vi "TankFill.vi"() -> ()   [LabVIEW 2018]
panel:
  out "?":string
  out "Min. Level":bool
  out "Max. Level":bool
  in  "Decrement/0.1sec":dbl(knob) scale=0.0..10.0
  in  "Increment/0.1sec":dbl(knob) scale=0.0..10.0
  in  "Min level":dbl(knob) scale=0.0..100.0
  in  "Max level":dbl(knob) scale=0.0..100.0
  out "Tank":dbl(slide) scale=0.0..100.0
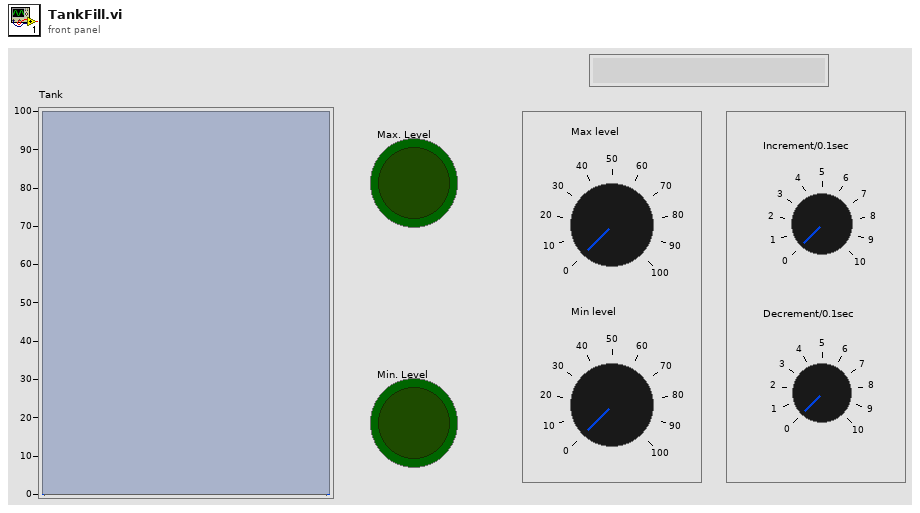
[diagram p1: front panel]
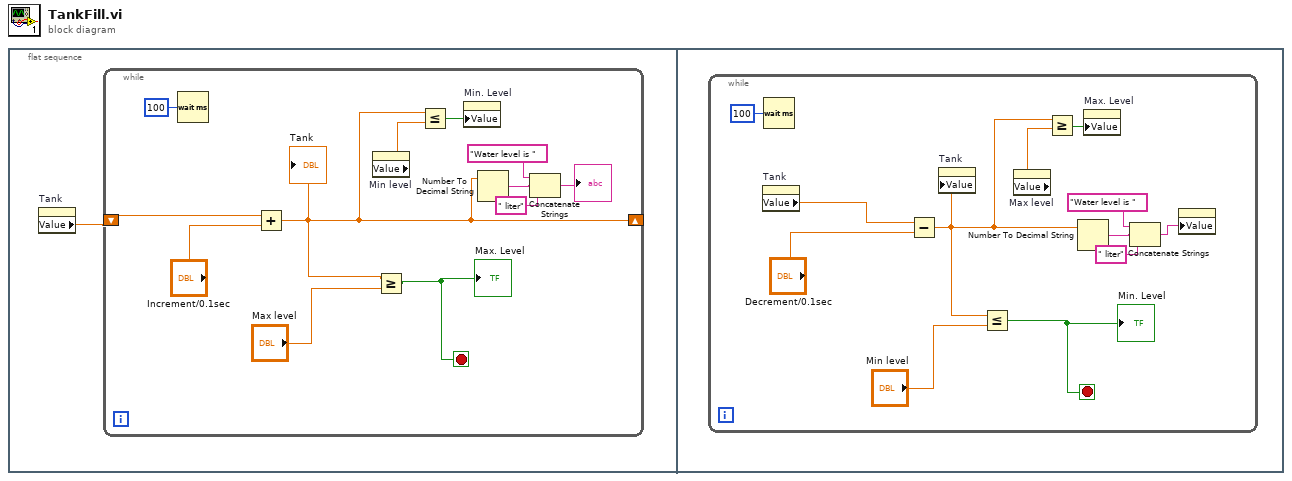
[diagram p0: block diagram]
diagram:
  n1 = flat-sequence {
    frame #0 {
      n2 = property on="Tank" class="Slide (strict)"() -> ("Value"=w1:dbl)  [unwired: 2 in, 2 out]
      n3 = while {
        shift-right: [w6] -> _
        shift-left: w1 -> [w13]
        stop <- w9 stop-if-true
        n4 = Wait (ms)(milliseconds to wait=u32 100) -> ()  [unwired: 1 out]
        n5 = Add(x=w13, y="Increment/0.1sec") -> (x+y=w6:dbl)
        "Tank" <- w6
        n6 = property on="Min level" class="Knob (strict)"() -> ("Value"=w7:dbl)  [unwired: 2 in, 2 out]
        n7 = Greater Or Equal?(x=w6, y="Max level") -> (x >= y?=w9:bool)
        "Max. Level" <- w9
        n8 = Less Or Equal?(x=w6, y=w7) -> (x <= y?=w8:bool)
        n9 = property on="Min. Level" class="Bool (strict)"("Value"=w8) -> ()  [unwired: 2 in, 2 out]
        n10 = Number To Decimal String(number=w6) -> (decimal integer string=w5:string)  [unwired: 1 in]
        n11 = Concatenate Strings("Water level is " ("string"), w5, " liter" ("string")) -> (→"?":string)
      }
    }
    frame #1 {
      n12 = while {
        stop <- w22 stop-if-true
        n13 = property on="Tank" class="Slide (strict)"() -> ("Value"=w15:dbl)  [unwired: 2 in, 2 out]
        n14 = Wait (ms)(milliseconds to wait=u32 100) -> ()  [unwired: 1 out]
        n15 = Subtract(x=w15, y="Decrement/0.1sec") -> (x-y=w14:dbl)
        n16 = property on="Tank" class="Slide (strict)"("Value"=w14) -> ()  [unwired: 2 in, 2 out]
        n17 = Less Or Equal?(x=w14, y="Min level") -> (x <= y?=w22:bool)
        "Min. Level" <- w22
        n18 = property on="Max level" class="Knob (strict)"() -> ("Value"=w20:dbl)  [unwired: 2 in, 2 out]
        n19 = Greater Or Equal?(x=w14, y=w20) -> (x >= y?=w21:bool)
        n20 = Number To Decimal String(number=w14) -> (decimal integer string=w19:string)  [unwired: 1 in]
        n21 = property on="Max. Level" class="Bool (strict)"("Value"=w21) -> ()  [unwired: 2 in, 2 out]
        n22 = Concatenate Strings("Water level is " ("string"), w19, " liter" ("string")) -> (w17:string)
        n23 = property class="Str"("Value"=w17) -> ()  [unwired: 2 in, 2 out]
      }
    }
  }
